vi "Read Results from processing.vi"(8 "error in":errorcluster, 11 "AppStateMachine runtime in":refnum<class "AppStateMachine runtime.lvclass">) -> (0 "error out":errorcluster, 2 "Results from processing":T1, 3 "AppStateMachine runtime out":refnum<class "AppStateMachine runtime.lvclass">)   [LabVIEW 2017, in "AppStateMachine runtime.lvclass"]
uses:
  AppStateMachine runtime.lvclass
  configuration/result data indices.ctl
  AppStateMachine runtime.lvclass/AppStateMachine runtime.ctl
  configuration/AppStateMachine configuration.lvclass
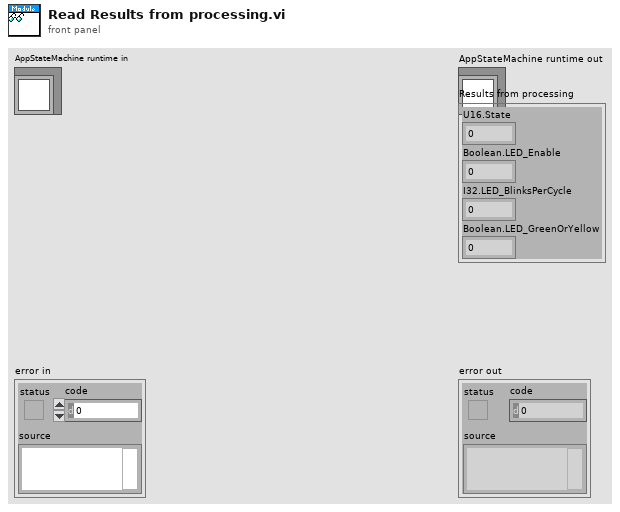
[diagram p1: front panel]
types:
  T1 = typedef "AppStateMachine configuration.lvclass/result data indices.ctl" = cluster{"U16.State":i32, "Boolean.LED_Enable":i32, "I32.LED_BlinksPerCycle":i32, "Boolean.LED_GreenOrYellow":i32}
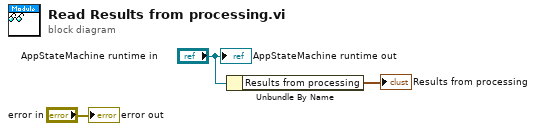
[diagram p0: block diagram]
diagram:
  n1 = Unbundle By Name("AppStateMachine runtime in") -> ("Results from processing"=→"Results from processing":T1)
  "error out" <- "error in"
  "AppStateMachine runtime out" <- "AppStateMachine runtime in"
